vi "Binary Instrument.vi"() -> ()   [LabVIEW 2019]
uses:
  <vilib>/Instr/_visa.llb/VISA Configure Serial Port (Instr).vi
panel:
  in  "Send":bool
  out "Max & Min":dbl[](array[numeric])
  out "error out":errorcluster
  in  "stop":bool
  in  "VISA resource name":refnum<visa-resource-name>
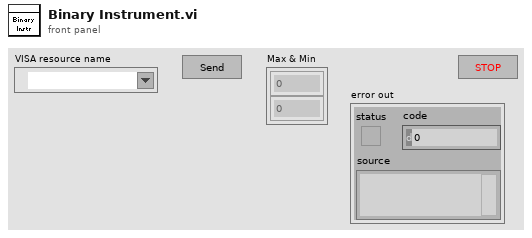
[diagram p1: front panel]
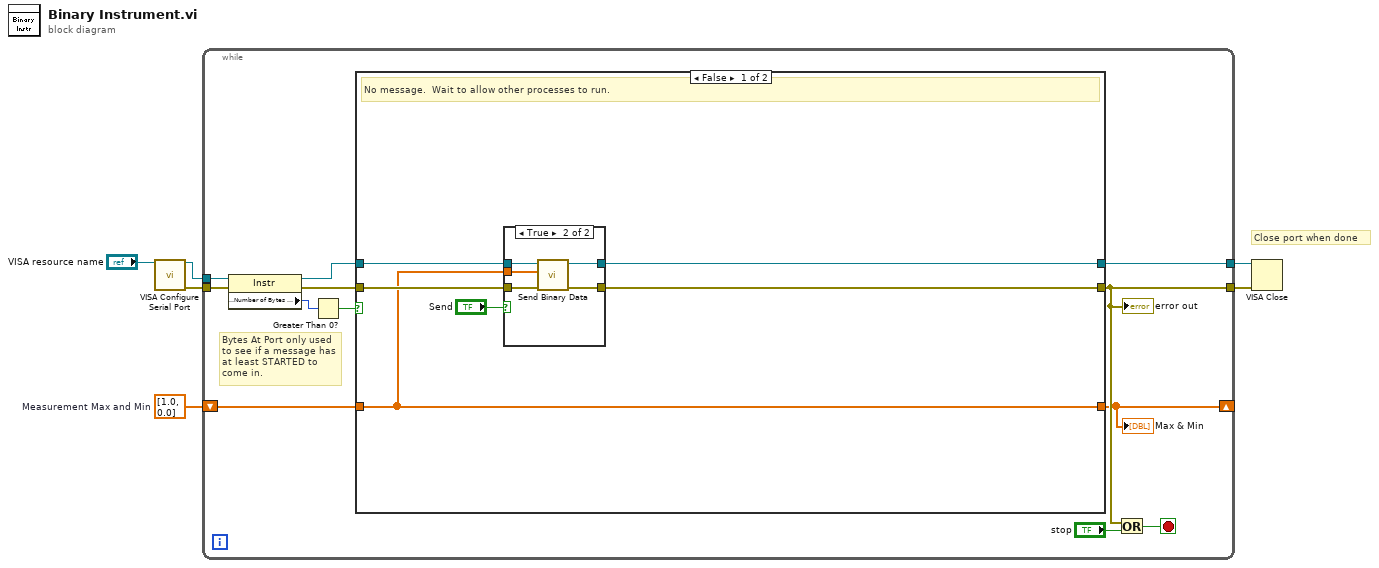
[diagram p0: block diagram]
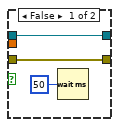
[diagram p2: hidden frame]
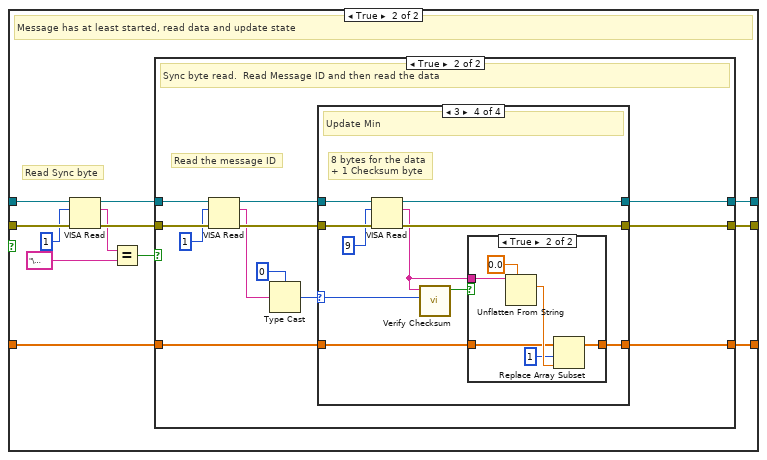
[diagram p3: hidden frame]
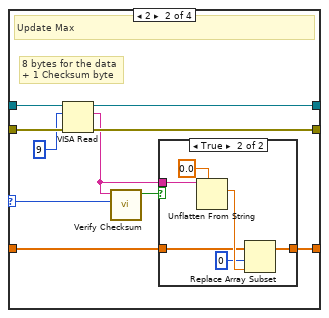
[diagram p6: hidden frame]
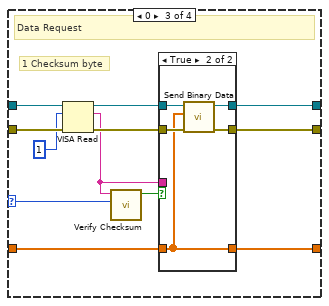
[diagram p8: hidden frame]
diagram:
  w2 = dbl[] [1.0, 0.0]  # Measurement Max and Min
  # "Close port when done"
  n1 = call-poly "VISA Configure Serial Port"("VISA resource name"="VISA resource name") -> ("VISA resource name out"=w1:refnum<visa-resource-name>, "error out"=w5:errorcluster)  [unwired: 13 in]
  n2 = while {
    tunnel: w5 -> [w18]
    tunnel: w1 -> [w15]
    tunnel: [w11] -> w3
    tunnel: [w16] -> w6
    shift-right: [w7] -> _
    shift-left: w2 -> [w8]
    stop <- w10 stop-if-true
    # "Bytes At Port only used\nto see if a message has\nat least STARTED to\ncome in."
    n3 = property class="Instr"(reference=w15, error in=w18) -> (reference out=w12:refnum<visa-resource-name>, error out=w17:errorcluster, "Serial Settings:Number of Bytes at Serial Port"=w14:u32)
    n4 = Greater Than 0?(x=w14) -> (x > 0?=w13:bool)
    n5 = case shown="False" w13 {
      tunnel: w17 -> [w22 w44]
      tunnel: w12 -> [w24 w41]
      tunnel: [w23 w33] -> w11
      tunnel: [w21 w42] -> w16
      tunnel: w8 -> [w20 w35]
      tunnel: [w20 w34] -> w7
      frame False {
        # "No message.  Wait to allow other processes to run."
        n6 = case shown="True" "Send" {
          tunnel: w24 -> [w26 w32]
          tunnel: [w26 w31] -> w23
          tunnel: w22 -> [w25 w30]
          tunnel: [w25 w29] -> w21
          tunnel: w20 -> [_ w28]
          frame False {
            n7 = Wait (ms)(milliseconds to wait=u32 50) -> ()  [unwired: 1 out]
          }
          frame True {
            n8 = call "Send Binary Data.vi"("error in"=w30, "Measurement Max and Min"=w28, "VISA Refnum in"=w32) -> ("error out"=w29:errorcluster, "VISA Refnum out"=w31:refnum<visa-resource-name>)  [unwired: 7 in]
          }
        }
      }
      frame True {
        # "Read Sync byte"
        # "Message has at least started, read data and update state"
        n9 = VISA Read(VISA resource name=w41, byte count=u32 1, error in (no error)=w44) -> (VISA resource name out=w37:refnum<visa-resource-name>, read buffer=w36:string, error out=w43:errorcluster)  [unwired: 1 out]
        n10 = Equal?(x=w36, y="\u0002") -> (x = y?=w38:bool)
        n11 = case shown="True" w38 {
          tunnel: w37 -> [w46 w55]
          tunnel: w43 -> [w47 w59]
          tunnel: [w46 w50] -> w33
          tunnel: [w47 w57] -> w42
          tunnel: w35 -> [w45 w49]
          tunnel: [w45 w48] -> w34
          frame False {
            # "Sync byte was not read.  Ignore the data assuming we are in the middle of a message."
          }
          frame True {
            # "Read the message ID"
            # "Sync byte read.  Read Message ID and then read the data"
            n12 = VISA Read(VISA resource name=w55, byte count=u32 1, error in (no error)=w59) -> (VISA resource name out=w51:refnum<visa-resource-name>, read buffer=w54:string, error out=w58:errorcluster)  [unwired: 1 out]
            n13 = Type Cast(type=u8 0, x=w54) -> (*(type *) &x=w52:u8)
            n14 = case shown="3" w52 {
              selector: w52 -> [_ w66 w85 w103]
              tunnel: w58 -> [w62 w72 w91 w109]
              tunnel: w51 -> [w61 w70 w88 w107]
              tunnel: [w61 w68 w80 w105] -> w50
              tunnel: [w62 w71 w89 w108] -> w57
              tunnel: w49 -> [w60 w64 w83 w101]
              tunnel: [w60 w63 w82 w100] -> w48
              frame Default {
                # "Unknown ID.  Ignore the data"
              }
              frame 2 {
                # "8 bytes for the data\n+ 1 Checksum byte"
                # "Update Max"
                n15 = VISA Read(VISA resource name=w70, byte count=u32 9, error in (no error)=w72) -> (VISA resource name out=w68:refnum<visa-resource-name>, read buffer=w65:string, error out=w71:errorcluster)  [unwired: 1 out]
                n16 = call "Verify Checksum.vi"("Message ID"=w66, "Data + Checksum"=w65) -> ("Pass"=w67:bool)  [unwired: 9 in]
                n17 = case shown="True" w67 {
                  tunnel: w65 -> [_ w78]
                  tunnel: w64 -> [w73 w75]
                  tunnel: [w73 w74] -> w63
                  frame False {
                  }
                  frame True {
                    n18 = Unflatten From String(type=0.0, binary string=w78) -> (value=w79:dbl)  [unwired: 3 in, 2 out]
                    n19 = Replace Array Subset(array=w75, new element=w79, index=0) -> (w74:dbl[])
                  }
                }
              }
              frame 0 {
                # "1 Checksum byte"
                # "Data Request"
                n20 = VISA Read(VISA resource name=w88, byte count=u32 1, error in (no error)=w91) -> (VISA resource name out=w81:refnum<visa-resource-name>, read buffer=w84:string, error out=w90:errorcluster)  [unwired: 1 out]
                n21 = call "Verify Checksum.vi"("Message ID"=w85, "Data + Checksum"=w84) -> ("Pass"=w86:bool)  [unwired: 9 in]
                n22 = case shown="True" w86 {
                  tunnel: w84 -> [_ _]
                  tunnel: w83 -> [w93 w96]
                  tunnel: [w93 w96] -> w82
                  tunnel: w81 -> [w92 w97]
                  tunnel: w90 -> [w94 w99]
                  tunnel: [w94 w98] -> w89
                  tunnel: [w92 w95] -> w80
                  frame False {
                  }
                  frame True {
                    n23 = call "Send Binary Data.vi"("error in"=w99, "Measurement Max and Min"=w96, "VISA Refnum in"=w97) -> ("error out"=w98:errorcluster, "VISA Refnum out"=w95:refnum<visa-resource-name>)  [unwired: 7 in]
                  }
                }
              }
              frame 3 {
                # "8 bytes for the data\n+ 1 Checksum byte"
                # "Update Min"
                n24 = VISA Read(VISA resource name=w107, byte count=u32 9, error in (no error)=w109) -> (VISA resource name out=w105:refnum<visa-resource-name>, read buffer=w102:string, error out=w108:errorcluster)  [unwired: 1 out]
                n25 = call "Verify Checksum.vi"("Message ID"=w103, "Data + Checksum"=w102) -> ("Pass"=w104:bool)  [unwired: 9 in]
                n26 = case shown="True" w104 {
                  tunnel: w102 -> [_ w115]
                  tunnel: w101 -> [w110 w112]
                  tunnel: [w110 w111] -> w100
                  frame False {
                  }
                  frame True {
                    n27 = Unflatten From String(type=0.0, binary string=w115) -> (value=w116:dbl)  [unwired: 3 in, 2 out]
                    n28 = Replace Array Subset(array=w112, new element=w116, index=1) -> (w111:dbl[])
                  }
                }
              }
            }
          }
        }
      }
    }
    "error out" <- w16
    "Max & Min" <- w7
    n29 = Or(x=w16, y="stop") -> (x .or. y?=w10:bool)
  }
  n30 = VISA Close(VISA resource name=w3, error in (no error)=w6) -> ()  [unwired: 1 out]
